vi "Set Mode Code.vi"(8 "error in":errorcluster, 10 "mode code":u16, 11 "message or subaddress":T1 format="%.0x") -> (0 "error out":errorcluster, 3 "message or subaddress out":T1 format="%.0x")   [LabVIEW 2020, in "AIM MIL-STD-1553 Scripting.lvlib"]
doc: "Sets the <b>mode code</b> for the input <b>message or subaddress</b>."
uses:
  AIM MIL-STD-1553 Scripting.lvlib
  <vilib>/NI VeriStand/Custom Device API/Custom Device Item Ref.ctl
  Constants.vi
  <vilib>/NI VeriStand/Custom Device API/Set Item Property (U16).vi
  <vilib>/NI VeriStand/Custom Device API/Custom Device API.lvlib
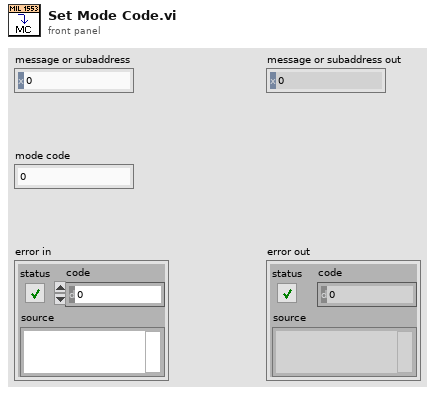
[diagram p1: front panel]
types:
  T1 = typedef "Custom Device API.lvlib/Custom Device Item Ref.ctl" = u64
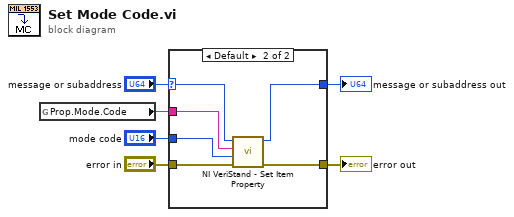
[diagram p0: block diagram]
diagram:
  n1 = global read "Constants.vi" "Prop.Mode.Code"() -> (w1:string)
  n2 = case shown="Default" "message or subaddress" {
    selector: "message or subaddress" -> [w8 w14]
    tunnel: [w8 w13] -> w5
    tunnel: "error in" -> [w7 w12]
    tunnel: [w7 w11] -> w3
    tunnel: "mode code" -> [_ w10]
    tunnel: w1 -> [_ w9]
    frame 0, -1 {
    }
    frame Default {
      n3 = call-poly <vilib>:"NI VeriStand - Set Item Property.vi"("error in (no error)"=w12, "Value"=w10, "Property Name"=w9, "Item Ref in"=w14) -> ("error out"=w11:errorcluster, "Item Ref out"=w13:T1)  [unwired: 5 in, 1 out]
    }
  }
  "message or subaddress out" <- w5
  "error out" <- w3
